vi "Release.vi"(8 "error in (no error)":errorcluster, 11 "MultiErrors in":refnum<class "MultiErrors.lvclass">) -> (0 "error out":errorcluster, 2 "Entries":T1[](array[typedef]))   [LabVIEW 2020, in "Volatus.lvlib" / "MultiErrors.lvclass"]
uses:
  MultiErrors.lvclass
  MultiError Entry.ctl
  MultiErrors.lvclass/MultiErrors.ctl
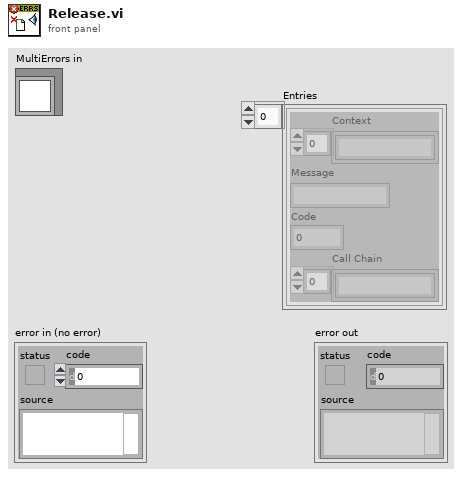
[diagram p1: front panel]
types:
  T1 = typedef "Volatus.lvlib/MultiErrors.lvclass/MultiError Entry.ctl" = cluster{"Context":string[], "Message":string, "Code":i32, "Call Chain":string[]}
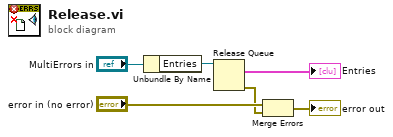
[diagram p0: block diagram]
diagram:
  n1 = Unbundle By Name("MultiErrors in") -> ("Entries"=w4:refnum<queue>)
  n2 = Release Queue(queue=w4) -> (remaining elements=→"Entries":T1[], error out=w1:errorcluster)  [unwired: 2 in, 1 out]
  n3 = Merge Errors("error in (no error)", w1) -> (→"error out":errorcluster)
